vi "Demo (Reference).vi"() -> ()   [LabVIEW 2010]
uses:
  <vilib>/MDSplus/Library/MDSplus.lvlib
panel:
  out "Waveform Graph 2":sgl[](graph)
  out "Waveform Graph":dynamicdata(graph)
  in  "stop":bool
  in  "Path":string=":SIG_0"
  in  "Shot":i32=-1
  in  "Name":string="my_tree"
  in  "sampling info":cluster{"Fs":dbl, "#s":dbl}={"Fs"=1000.0, "#s"=1000.0}
  in  "phase":dbl
  in  "amplitude":dbl=5.0
  in  "frequency":dbl=1.1
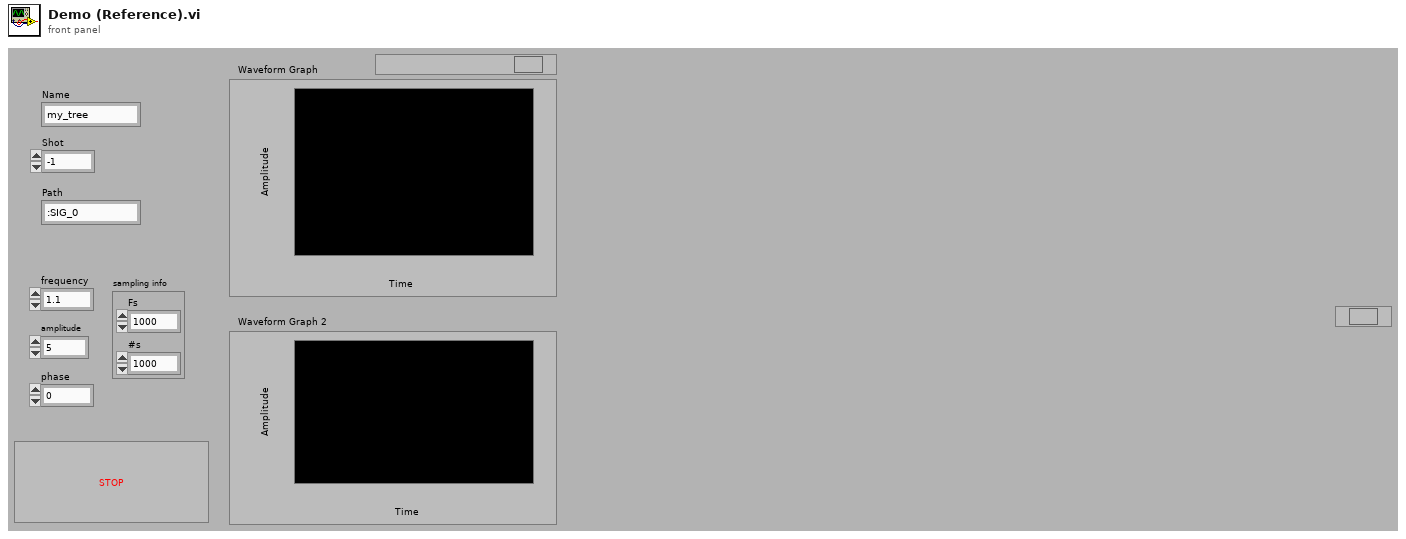
[diagram p1: front panel]
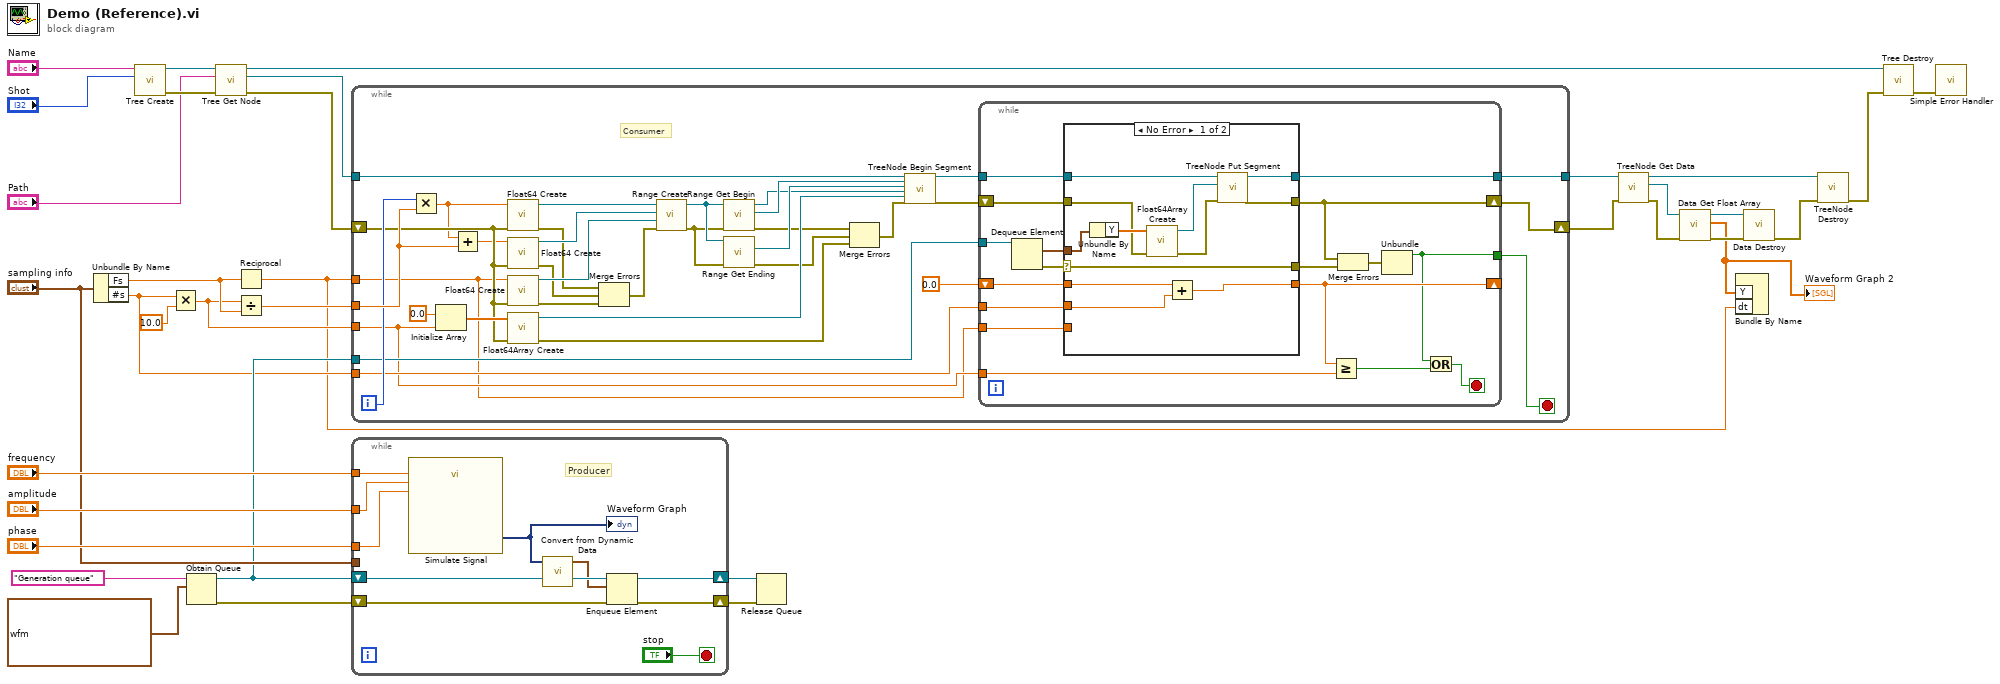
[diagram p0: block diagram]
diagram:
  n1 = Unbundle By Name("sampling info") -> ("Fs"=w30:dbl, "#s"=w18:dbl)
  n2 = call <vilib>:"Tree Create.vi"("Shot"="Shot", "Name"="Name") -> ("error out"=w34:errorcluster, "Tree DVR out"=w35:refnum<data-value>)  [unwired: 8 in]
  n3 = Multiply(x=w18, y=10.0) -> (x*y=w27:dbl)
  n4 = Obtain Queue(name (unnamed)="Generation queue", element data type=waveform(dbl) {"t0"=timestamp(0 s since 1904-01-01), "dt"=1.0, "Y"=[]} ("Waveform")) -> (queue out=w19:refnum<queue>, error out=w20:errorcluster)  [unwired: 3 in, 1 out]
  n5 = call <vilib>:"Tree Get Node.vi"("error in (no error)"=w34, "Path"="Path", "Tree DVR in"=w35) -> ("error out"=w12:errorcluster, "Node out"=w11:refnum<data-value>, "Tree DVR out"=w13:refnum<data-value>)  [unwired: 6 in]
  n6 = Reciprocal(x=w30) -> (1/x=w3:dbl)
  n7 = Divide(x=w27, y=w30) -> (x/y=w29:dbl)
  n8 = while {
    tunnel: w11 -> [w70]
    tunnel: [w60] -> w10
    tunnel: w3 -> [w38]
    tunnel: w29 -> [w55]
    tunnel: w27 -> [w41]
    tunnel: w19 -> [w50]
    shift-right: [w39] -> w8
    shift-left: w12 -> [w51]
    tunnel: w18 -> [w43]
    i -> [w53]
    stop <- w40 stop-if-true
    # "Consumer"
    n9 = Multiply(x=w53, y=w55) -> (x*y=w36:dbl)
    n10 = Initialize Array(0.0 ("element"), w41) -> (w52:dbl[])
    n11 = Add(x=w36, y=w55) -> (x+y=w37:dbl)
    n12 = call <vilib>:"Float64 Create.vi"("error in (no error)"=w51, "DBL in"=w36) -> ("error out"=w64:errorcluster, "Float64 DVR out"=w69:refnum<data-value>)  [unwired: 8 in]
    n13 = call <vilib>:"Float64 Create.vi"("error in (no error)"=w51, "DBL in"=w37) -> ("error out"=w66:errorcluster, "Float64 DVR out"=w68:refnum<data-value>)  [unwired: 8 in]
    n14 = call <vilib>:"Float64 Create.vi"("error in (no error)"=w51, "DBL in"=w38) -> ("error out"=w65:errorcluster, "Float64 DVR out"=w67:refnum<data-value>)  [unwired: 8 in]
    n15 = call <vilib>:"Float64Array Create.vi"("error in (no error)"=w51, "DBL array in"=w52) -> ("error out"=w57:errorcluster, "Float64Array DVR out"=w62:refnum<data-value>)  [unwired: 8 in]
    n16 = Merge Errors(w64, w66, w65) -> (w63:errorcluster)
    n17 = call <vilib>:"Range Create.vi"("error in (no error)"=w63, "Delta value"=w67, "Ending"=w68, "Begin"=w69) -> ("error out"=w47:errorcluster, "Range DVR out"=w48:refnum<data-value>)  [unwired: 6 in]
    n18 = call <vilib>:"Range Get Begin.vi"("error in (no error)"=w47, "Range DVR in"=w48) -> ("error out"=w45:errorcluster, "Begin out"=w59:refnum<data-value>, "Range DVR out"=w46:refnum<data-value>)  [unwired: 7 in]
    n19 = call <vilib>:"Range Get Ending.vi"("error in (no error)"=w47, "Range DVR in"=w48) -> ("error out"=w44:errorcluster, "Ending out"=w58:refnum<data-value>)  [unwired: 7 in, 1 out]
    n20 = Merge Errors(w45, w44, w57) -> (w56:errorcluster)
    n21 = call <vilib>:"TreeNode Begin Segment.vi"("TreeNode DVR in"=w70, "Start"=w59, "End"=w58, "Dimension"=w46, "Initial data"=w62, "error in (no error)"=w56) -> ("TreeNode DVR out"=w61:refnum<data-value>, "error out"=w49:errorcluster)  [unwired: 12 in]
    n22 = while {
      tunnel: w61 -> [w87]
      tunnel: [w86] -> w60
      tunnel: w50 -> [w85]
      tunnel: w43 -> [w81]
      shift-right: [w80] -> _
      shift-left: 0.0 ("#s") -> [w82]
      tunnel: w41 -> [w79]
      shift-right: [w71] -> w39
      shift-left: w49 -> [w78]
      tunnel: [w73] -> w40
      tunnel: w38 -> [w72]
      stop <- w76 stop-if-true
      n23 = Dequeue Element(queue=w85) -> (element=w84:waveform(dbl), error out=w83:errorcluster)  [unwired: 2 in, 2 out]
      n24 = case shown="No Error" w83 {
        selector: w83 -> [w93 w102]
        tunnel: w87 -> [w99 w103]
        tunnel: [w89 w103] -> w86
        tunnel: w84 -> [w95 _]
        tunnel: [w93 w102] -> w75
        tunnel: w82 -> [w91 w101]
        tunnel: w81 -> [w92 _]
        tunnel: [w90 w101] -> w80
        tunnel: [w88 w100] -> w71
        tunnel: w78 -> [w94 w100]
        tunnel: w72 -> [_ _]
        frame No Error {
          n25 = Unbundle By Name(w95) -> ("Y"=w98:dbl[])
          n26 = call <vilib>:"Float64Array Create.vi"("error in (no error)"=w94, "DBL array in"=w98) -> ("error out"=w97:errorcluster, "Float64Array DVR out"=w96:refnum<data-value>)  [unwired: 8 in]
          n27 = Add(x=w91, y=w92) -> (x+y=w90:dbl)
          n28 = call <vilib>:"TreeNode Put Segment.vi"("error in (no error)"=w97, "Data"=w96, "TreeNode DVR in"=w99) -> ("error out"=w88:errorcluster, "TreeNode DVR out"=w89:refnum<data-value>)  [unwired: 7 in]
        }
        frame Error {
          # "Producer stopped"
        }
      }
      n29 = Greater Or Equal?(x=w80, y=w79) -> (x >= y?=w77:bool)
      n30 = Merge Errors(w71, w75) -> (w74:errorcluster)
      n31 = Unbundle(w74) -> ("status"=w73:bool)  [unwired: 2 out]
      n32 = Or(x=w73, y=w77) -> (x .or. y?=w76:bool)
    }
  }
  n33 = while {
    tunnel: "frequency" -> [w108]
    tunnel: "amplitude" -> [w107]
    tunnel: "phase" -> [w106]
    tunnel: "sampling info" -> [_]
    shift-right: [w111] -> w17
    shift-left: w19 -> [w113]
    shift-right: [w110] -> w16
    shift-left: w20 -> [w112]
    stop <- "stop" stop-if-true
    # "Producer"
    n34 = call "Simulate Signal"("Frequency"=w108, "Amplitude"=w107, "Phase"=w106) -> ("Sine with Uniform Noise"=w105:dynamicdata)  [unwired: 11 in, 1 out]
    "Waveform Graph" <- w105
    n35 = call "Convert from Dynamic Data"("Dynamic Data Type"=w105) -> ("Waveform"=w104:waveform(dbl))  [unwired: 3 in]
    n36 = Enqueue Element(queue=w113, element=w104, error in (no error)=w112) -> (queue out=w111:refnum<queue>, error out=w110:errorcluster)  [unwired: 1 in, 1 out]
  }
  n37 = Release Queue(queue=w17, error in (no error)=w16) -> ()  [unwired: 1 in, 3 out]
  n38 = call <vilib>:"TreeNode Get Data.vi"("error in (no error)"=w8, "TreeNode DVR in"=w10) -> ("error out"=w6:errorcluster, "Data out"=w7:refnum<data-value>, "TreeNode DVR out"=w9:refnum<data-value>)  [unwired: 7 in]
  n39 = call <vilib>:"Data Get Float Array.vi"("error in (no error)"=w6, "Data DVR in"=w7) -> ("error out"=w5:errorcluster, "SGL array out"=w1:sgl[], "Data DVR out"=w4:refnum<data-value>)  [unwired: 6 in, 1 out]
  "Waveform Graph 2" <- w1
  n40 = Bundle By Name("Y"=w1, "dt"=w3) -> ()  [unwired: 1 in, 1 out]
  n41 = call <vilib>:"Data Destroy.vi"("error in (no error)"=w5, "Data DVR in"=w4) -> ("error out"=w2:errorcluster)  [unwired: 9 in]
  n42 = call <vilib>:"TreeNode Destroy.vi"("error in (no error)"=w2, "TreeNode DVR in"=w9) -> ("error out"=w14:errorcluster)  [unwired: 9 in]
  n43 = call <vilib>:"Tree Destroy.vi"("error in (no error)"=w14, "Tree DVR in"=w13) -> ("error out"=w15:errorcluster)  [unwired: 9 in]
  n44 = call <vilib>:"Simple Error Handler.vi"("error in (no error)"=w15) -> ()  [unwired: 4 in, 5 out]
